vi "Hang Controller.vi"(8 "error in":errorcluster) -> ()   [LabVIEW 2019]
doc: "This VI executes continuously carrying out the current operation and responding to updates or new operations. It will often contain the timing or control code that is difficult to place directly in TeleOp. This VI generally opens all sensors and motors and isolates the rest of the robot code from knowing how the operations are carried out."
uses:
  <vilib>/Rock Robotics/WPI/Framework/Completion Status.ctl
  Hang Setpoints.ctl
  Hang Operations.ctl
  <vilib>/Rock Robotics/SystemInterfaces/DIO/FPGA_DIOPWMChannel.ctl
  <vilib>/Rock Robotics/WPI/ThirdParty/Phoenix-LabVIEW/Motor Controller/Controls/CTRE_Phoenix_MotorControl_ControlMode.ctl
  <vilib>/Rock Robotics/WPI/ThirdParty/Phoenix-LabVIEW/Motor Controller/Get/CTRE_Phoenix_MotorController_GetSelectedSensorData.vi
  <vilib>/Rock Robotics/Network Tables/NT Write Boolean.vi
panel:
  in  "Output":dbl
  in  "servo position":dbl
  out "sensor pos":i32
  in  "Position":dbl
  in  "Interactive Values":T1
  out "Current\nCmd":string
  in  "Buttons":cluster{"Execute Cmd":bool, "Abort Cmd":bool}
  out "Command Timing":cluster{"Start Time (ms)":u32, "Iterations":i32}
  out "Status":T3
  # "Tip: It may be helpful to observe inputs and sensor values.\nYou may also want to display tuning or debugging controls."
  # "Interactive Command: You may fill in the settings for a command\nand schedule it with the Execute button. You can observe and abort\nany command while fine tuning the code for the controller."
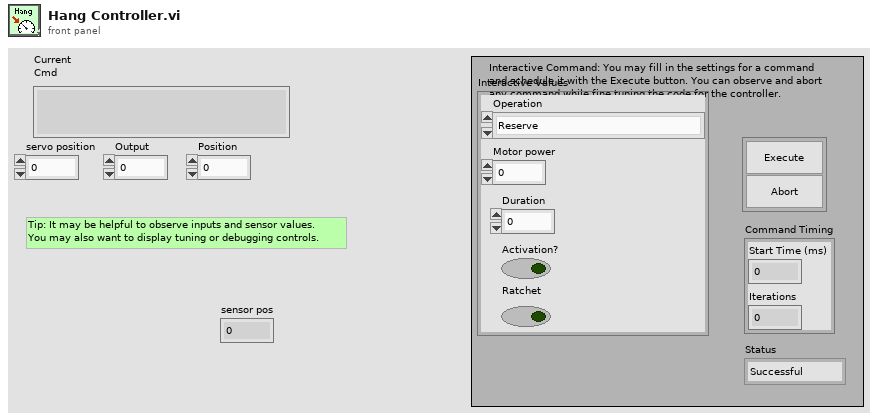
[diagram p1: front panel]
types:
  T1 = typedef "Hang Setpoints.ctl" = cluster{"Operation":T2, "Motor power":dbl, "Activation?":bool, "Ratchet":bool, "Duration":dbl}
  T2 = typedef "Hang Operations.ctl" = enum16{"Reserve", "Read Current", "Immediate", "Undo Servo"}
  T3 = typedef "Completion Status.ctl" = enum16{"Successful", "Aborted", "Incomplete"}
  T4 = typedef "FPGA_DIOPWMChannel.ctl" = enum8{"PWM 0", "PWM 1", "PWM 2", "PWM 3", "PWM 4", "PWM 5", "PWM 6", "PWM 7", "PWM 8", "PWM 9", "PWM MXP 0", "PWM MXP 1", "PWM MXP 2", "PWM MXP 3", "PWM MXP 4", "PWM MXP 5", "PWM MXP 6", "PWM MXP 7", "PWM MXP 8", "PWM MXP 9", "Invalid"}
  T5 = typedef "WPI_MotorControlDeviceRef.ctl" = cluster{"DeviceStatus":errorcluster, "Type":T6, "PWM":cluster{"PWM Channel":T4, "DeadBand":T7}, "CAN":cluster{"Device Number":u8, "SetOutput VI Ref":variant, "GetOutput VI Ref":variant, "Enable VI Ref":variant, "Disable VI Ref":variant, "Data":variant}, "Invert":bool, "DIO PWM":cluster{"PWM \"Enable\" Channel":T4, "DIOChannel":T8, "PWM Rate":dbl}}
  T6 = typedef "WPI_MotorControlType.ctl" = enum16{"PWM", "CAN", "DIO PWM"}
  T7 = typedef "WPI_PWMDeadband.ctl" = cluster{"Name":string, "maxPositivePwm":i32, "minPositivePwm":i32, "centerPwm":i32, "maxNegativePwm":i32, "minNegativePwm":i32, "angularRange":u16}
  T8 = typedef "FPGA_DIOChannel.ctl" = enum8{"DIO 0", "DIO 1", "DIO 2", "DIO 3", "DIO 4", "DIO 5", "DIO 6", "DIO 7", "DIO 8", "DIO 9", "DIO MXP 0", "DIO MXP 1", "DIO MXP 2", "DIO MXP 3", "DIO MXP 4", "DIO MXP 5", "DIO MXP 6", "DIO MXP 7", "DIO MXP 8", "DIO MXP 9", "DIO MXP 10", "DIO MXP 11", "DIO MXP 12", "DIO MXP 13", "DIO MXP 14", "DIO MXP 15", "SPI Port CS1", "SPI Port CS2", "SPI Port CS3", "SPI Port MISO", "SPI Port MOSI", "Invalid"}
  T9 = typedef "WPI_ServoDeviceRef.ctl" = cluster{"DeviceStatus":errorcluster, "PWM Channel":T4, "DeadBand":T7}
  T10 = typedef "Command Status Info.ctl" = cluster{"Name":string, "Status":T3, "notifier out":T11}
  T11 = typedef "Completion Notifier.ctl" = refnum<notifier>
  T12 = cluster{"Current Command":T1, "Command Timing":cluster{"Start Time (ms)":u32, "Iterations":i32}, "Command Arguments":cluster{"Command Info":T10, "Description":string, "Default Command":T1, "queue out":refnum<queue>, "Subsystem Name":string}}
  T13 = typedef "CTRE_Phoenix_MotorControl_ControlMode.ctl" = u16
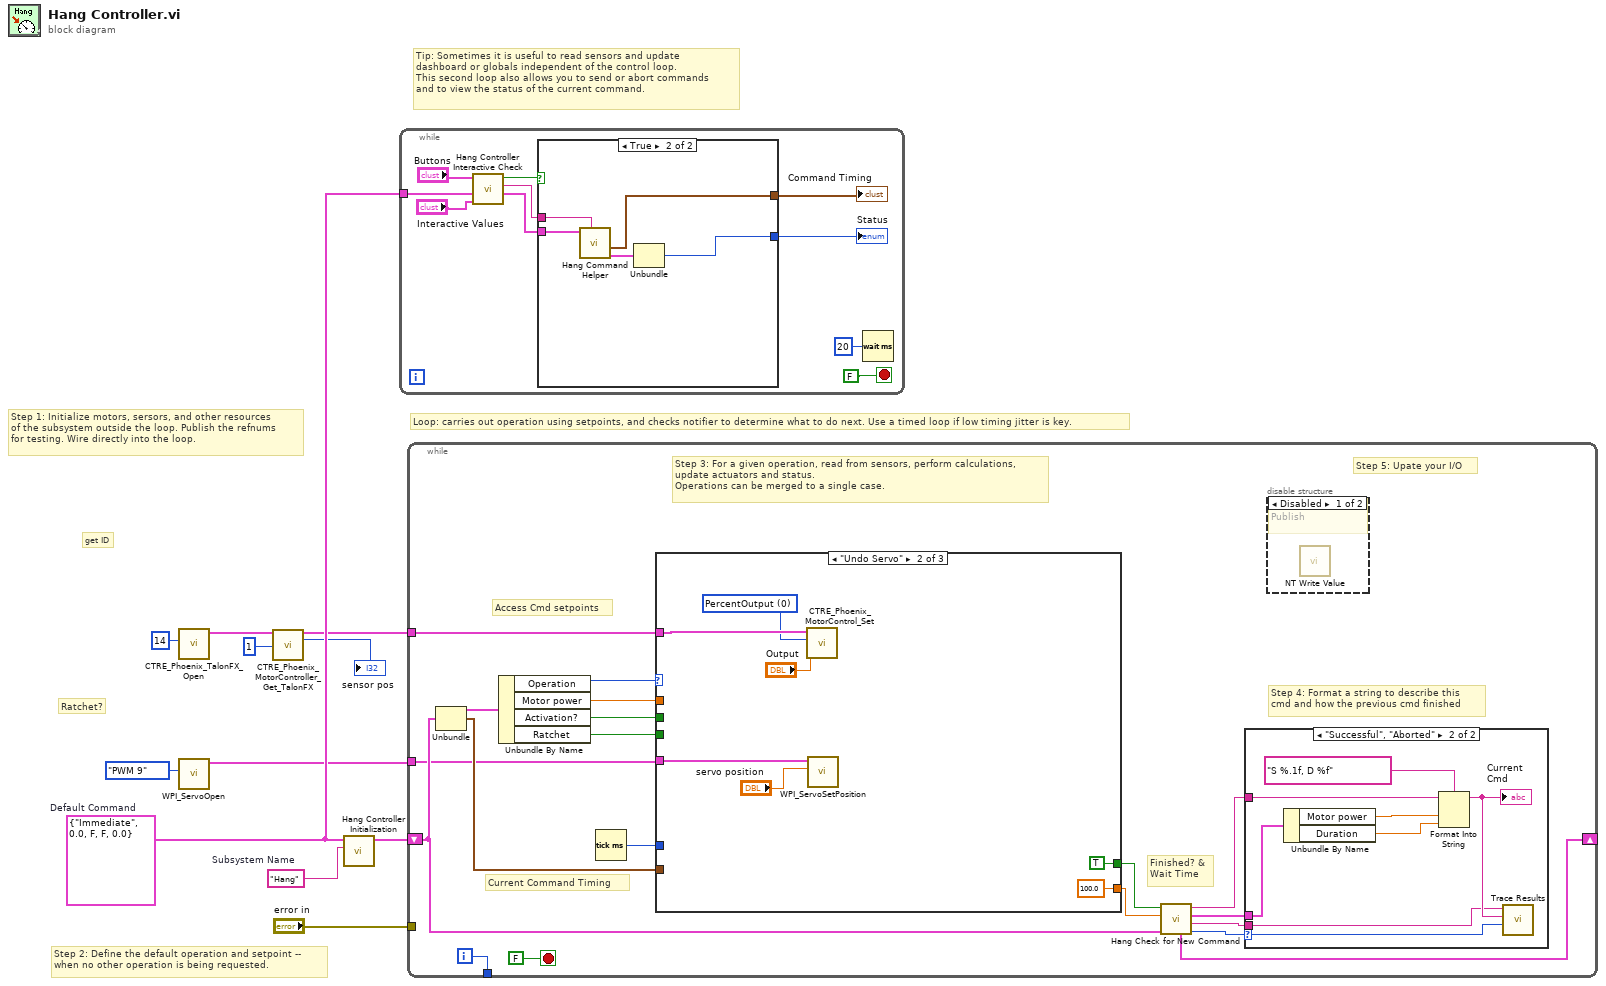
[diagram p0: block diagram]
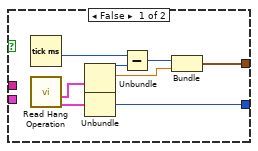
[diagram p2: hidden frame]
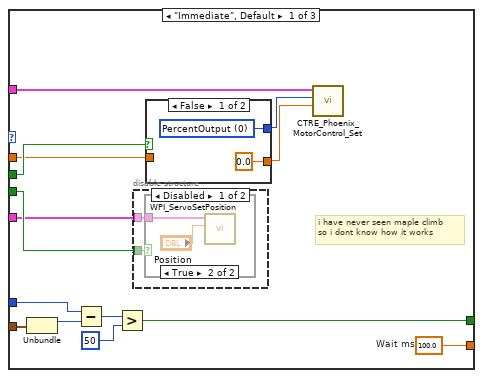
[diagram p5: hidden frame]
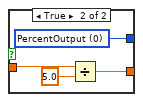
[diagram p8: hidden frame]
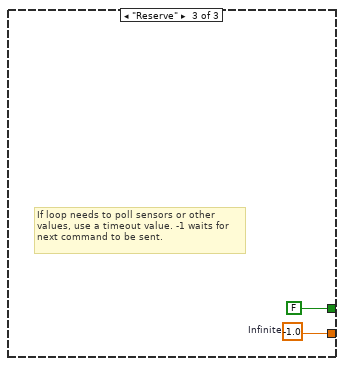
[diagram p9: hidden frame]
diagram:
  w8 = T1 {"Operation"=enum."Immediate", "Motor power"=0.0, "Activation?"=FALSE, "Ratchet"=FALSE, "Duration"=0.0}  # Default Command
  w9 = "Hang"  # Subsystem Name
  # "get ID"
  # "Ratchet?"
  # "Tip: Sometimes it is useful to read sensors and update\ndashboard or globals independent of the control loop.\nThis second loop also allows you to send or abort commands\nand to view the status of the current command."
  # "Step 2: Define the default operation and setpoint --\nwhen no other operation is being requested."
  # "Step 1: Initialize motors, sersors, and other resources\nof the subsystem outside the loop. Publish the refnums\nfor testing. Wire directly into the loop."
  # "Loop: carries out operation using setpoints, and checks notifier to determine what to do next. Use a timed loop if low timing jitter is key."
  n1 = call <vilib>:"CTRE_Phoenix_TalonFX_Open.vi"("Device Number"=u8 14) -> ("CAN Talon SRX Ref"=w2:T5)  [unwired: 9 in, 1 out]
  n2 = call <vilib>:"WPI_ServoOpen.vi"("PWM Channel"=FPGA_DIOPWMChannel."PWM 9") -> ("ServoDeviceRef"=w5:T9)  [unwired: 9 in, 1 out]
  n3 = call-poly <vilib>:"CTRE_Phoenix_MotorController_Get_TalonFX.vi"("PhoenixMotorControlDevRef"=w2, "pidLoopIdx"=u32 1) -> ("PhoenixMotorControlDevRef"=w1:T5, "Position (Raw Sensor Units)"=→"sensor pos":i32)  [unwired: 10 in, 2 out]
  n4 = call "Hang Controller Initialization.vi"("Subsystem Name"=w9, "Default Command"=w8) -> ("Current Command"=w10:T12)  [unwired: 9 in]
  n5 = while {
    tunnel: w8 -> [w18]
    stop <- FALSE stop-if-true
    n6 = call "Hang Controller Interactive Check.vi"("Interactive Command in"="Interactive Values", "Default Command"=w18, "Buttons"="Buttons") -> ("Interactive Command out"=w15:T1, "Trace String"=w16:string, "Schedule"=w17:bool)  [unwired: 6 in]
    n7 = case shown="True" w17 {
      tunnel: [w29 w34] -> w14
      tunnel: w15 -> [_ w32]
      tunnel: [w25 w30] -> w13
      tunnel: w16 -> [_ w33]
      frame False {
        n8 = Tick Count (ms)() -> (millisecond timer value=w24:u32)
        n9 = call "Read Hang Operation.vi"() -> ("Command Info"=w22:T10, "SubSystem Data"=w23:T1)  [unwired: 9 in, 1 out]
        n10 = Unbundle(w23) -> ("Operation"=w28:T2, "Motor power"=w26:dbl)  [unwired: 3 out]
        n11 = Unbundle(w22) -> ("Status"=w29:T3)  [unwired: 2 out]
        n12 = Subtract(x=w24, y=w28) -> (x-y=w27:u32)
        n13 = Bundle(w27, "Motor power"=w26) -> (w25:cluster{u32, "Motor power":dbl})  [unwired: 1 in]
      }
      frame True {
        n14 = call "Hang Command Helper.vi"("Description"=w33, "SubSystem Data"=w32) -> ("Command Info Out"=w31:T10, "Command Timing"=w30:cluster{"Start Time (ms)":u32, "Iterations":i32})  [unwired: 7 in, 1 out]
        n15 = Unbundle(w31) -> ("Status"=w34:T3)  [unwired: 2 out]
      }
    }
    "Status" <- w14
    "Command Timing" <- w13
    n16 = Wait (ms)(milliseconds to wait=u32 20) -> ()  [unwired: 1 out]
  }
  n17 = while {
    shift-right: [w46] -> _
    shift-left: w10 -> [w39]
    tunnel: [w52] -> _
    tunnel: "error in" -> [_]
    tunnel: w5 -> [w35]
    tunnel: w1 -> [w36]
    i -> [w52]
    stop <- FALSE stop-if-true
    # "Step 5: Upate your I/O"
    # "Step 4: Format a string to describe this\ncmd and how the previous cmd finished"
    # "Current Command Timing"
    # "Access Cmd setpoints"
    # "Finished? &\nWait Time"
    # "Step 3: For a given operation, read from sensors, perform calculations,\nupdate actuators and status.\nOperations can be merged to a single case."
    n18 = Unbundle(w39) -> ("Current Command"=w51:T1, "Command Timing"=w48:cluster{"Start Time (ms)":u32, "Iterations":i32})  [unwired: 1 out]
    n19 = Unbundle By Name(w51) -> ("Operation"=w50:T2, "Motor power"=w38:dbl, "Activation?"=w47:bool, "Ratchet"=w37:bool)
    n20 = Tick Count (ms)() -> (millisecond timer value=w49:u32)
    n21 = case shown="\"Undo Servo\"" w50 {
      tunnel: [w75 100.0 ("Infinite") w94] -> w44
      tunnel: [w69 TRUE ("ignore previous (F)") FALSE ("ignore previous (F)")] -> w45
      tunnel: w48 -> [w71 _ _]
      tunnel: w49 -> [w70 _ _]
      tunnel: w47 -> [w65 _ _]
      tunnel: w38 -> [w64 _ _]
      tunnel: w37 -> [w68 _ _]
      tunnel: w36 -> [w63 w90 _]
      tunnel: w35 -> [w62 w92 _]
      frame "Immediate", Default {
        w75 = 100.0  # Wait ms
        # "i have never seen maple climb\nso i dont know how it works"
        n22 = Unbundle(w71) -> ("Start Time (ms)"=w74:u32)  [unwired: 1 out]
        n23 = Subtract(x=w70, y=w74) -> (x-y=w73:u32)
        n24 = Greater?(x=w73, y=u8 50 ("Left Motor")) -> (0:w69:bool)
        n25 = disable-structure shown="Disabled" {
          disable-tunnel: w68 -> [w77 _]
          disable-tunnel: w62 -> [w76 _]
          frame Disabled {
            n26 = case shown="True" w77 {
              tunnel: w76 -> [_ w78]
              frame False {
              }
              frame True {
                n27 = call <vilib>:"WPI_ServoSetPosition.vi"("Position"="Position", "ServoDeviceRef"=w78) -> ()  [unwired: 8 in, 2 out]
              }
            }
          }
          frame Enabled {
          }
        }
        n28 = case shown="False" w65 {
          tunnel: [w81 w85] -> w67
          tunnel: [0.0 ("Motor position") w82] -> w66
          tunnel: w64 -> [_ w83]
          frame False {
            w81 = T13 0 items=["PercentOutput"=0, "Position"=1, "Velocity"=2, "Current"=3, "Follower"=5, "MotionProfile"=6, "MotionMagic"=7, "MotionProfileArc"=10, "Disabled"=15] ("Control Mode")
          }
          frame True {
            w85 = T13 0 items=["PercentOutput"=0, "Position"=1, "Velocity"=2, "Current"=3, "Follower"=5, "MotionProfile"=6, "MotionMagic"=7, "MotionProfileArc"=10, "Disabled"=15] ("Control Mode")
            n29 = Divide(x=w83, y=5.0) -> (x/y=w82:dbl)
          }
        }
        n30 = call <vilib>:"CTRE_Phoenix_MotorControl_Set.vi"("Output"=w66, "Control Mode"=w67, "PhoenixMotorControlDevRef"=w63) -> ()  [unwired: 7 in, 2 out]
      }
      frame "Undo Servo" {
        w89 = T13 0 items=["PercentOutput"=0, "Position"=1, "Velocity"=2, "Current"=3, "Follower"=5, "MotionProfile"=6, "MotionMagic"=7, "MotionProfileArc"=10, "Disabled"=15] ("Control Mode")
        n31 = call <vilib>:"CTRE_Phoenix_MotorControl_Set.vi"("Output"="Output", "Control Mode"=w89, "PhoenixMotorControlDevRef"=w90) -> ()  [unwired: 7 in, 2 out]
        n32 = call <vilib>:"WPI_ServoSetPosition.vi"("Position"="servo position", "ServoDeviceRef"=w92) -> ()  [unwired: 8 in, 2 out]
      }
      frame "Reserve" {
        w94 = -1.0  # Infinite
        # "If loop needs to poll sensors or other\nvalues, use a timeout value. -1 waits for\nnext command to be sent."
      }
    }
    n33 = call "Hang Check for New Command.vi"("Current Command"=w39, "Wait time (ms)"=w44, "Finished?"=w45) -> ("Completion"=w40:T3, "Subsystem Name"=w41:string, "Current Command"=w42:T1, "Initial Trace String"=w43:string, "NextCommand"=w46:T12)  [unwired: 4 in]
    n34 = case shown="\"Successful\", \"Aborted\"" w40 {
      selector: w40 -> [_ w61]
      tunnel: w43 -> [_ w57]
      tunnel: w42 -> [_ w58]
      tunnel: w41 -> [_ w54]
      frame "Incomplete", Default {
        # "Continuing current command"
      }
      frame "Successful", "Aborted" {
        # "Report and setup for next command"
        n35 = Unbundle By Name(w58) -> ("Motor power"=w60:dbl, "Duration"=w55:dbl)
        n36 = Format Into String(format string="S %.1f, D %f", initial string=w57, w60, w55) -> (resulting string=w56:string)  [unwired: 1 in, 1 out]
        "Current\nCmd" <- w56
        n37 = call <vilib>:"Trace Results.vi"("Status of previous command"=w61, "Description"=w56, "Subsystem"=w54) -> ()  [unwired: 9 in]
      }
    }
    n38 = disable-structure shown="Disabled" {
      frame Disabled {
        # "Publish"
        n39 = call-poly <vilib>:"NT Write Value.vi"() -> ()  [unwired: 11 in, 1 out]
      }
      frame Enabled {
      }
    }
  }
